vi "WPI_JoystickGetInfo.vi"(8 "error in (no error)":errorcluster, 11 "JoystickDevice":T1) -> (0 "error out":errorcluster, 2 "Joystick Info":T2)   [LabVIEW 2017]
doc: "Returns name, type, axis information, button and POV count for a joystick that you specify.\n\nThis software is licensed. Open the labview\\readme\\WPI Robotics Library Open Source License.txt file for more information."
uses:
  <vilib>/Rock Robotics/WPI/Joystick/WPI_Joystick Info.ctl
  <vilib>/Rock Robotics/WPI/Joystick/WPI_JoystickHID Types.ctl
  <vilib>/Rock Robotics/WPI/Joystick/WPI_JoystickXBox Types.ctl
  <vilib>/Rock Robotics/WPI/Joystick/WPI_JoystickAxis Types.ctl
  <vilib>/Rock Robotics/WPI/Joystick/WPI_JoystickDeviceEnum.ctl
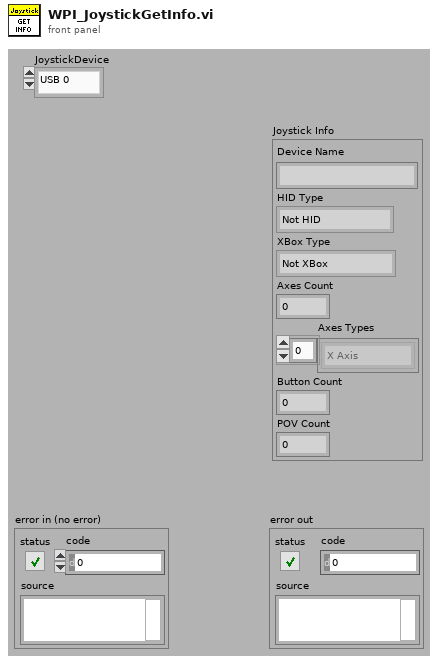
[diagram p1: front panel]
types:
  T1 = typedef "WPI_JoystickDeviceEnum.ctl" = enum16{"USB 0", "USB 1", "USB 2", "USB 3", "USB 4", "USB 5"}
  T2 = typedef "WPI_Joystick Info.ctl" = cluster{"Device Name":string, "HID Type":T3, "XBox Type":T4, "Axes Count":i32, "Axes Types":T5[], "Button Count":i32, "POV Count":i32}
  T3 = typedef "WPI_JoystickHID Types.ctl" = enum16{"Not HID", "HID Joystick", "HID Gamepad", "HID Driving Wheel", "HID Flightstick", "HID First Person"}
  T4 = typedef "WPI_JoystickXBox Types.ctl" = enum16{"Not XBox", "XBox Unknown", "XBox Gamepad", "XBox Wheel", "XBox Arcade Stick", "XBox Flight Stick", "XBox Dance Pad", "XBox Guitar", "XBox Drum Kit", "XBox Arcade Pad"}
  T5 = typedef "WPI_JoystickAxis Types.ctl" = enum16{"X Axis", "Y Axis", "Z Axis", "RxAxis", "RyAxis", "RzAxis", "Slider", "POV", "None", "L X Axis", "L Y Axis", "L Trigger", "R Trigger", "R X Axis", "R Y Axis"}
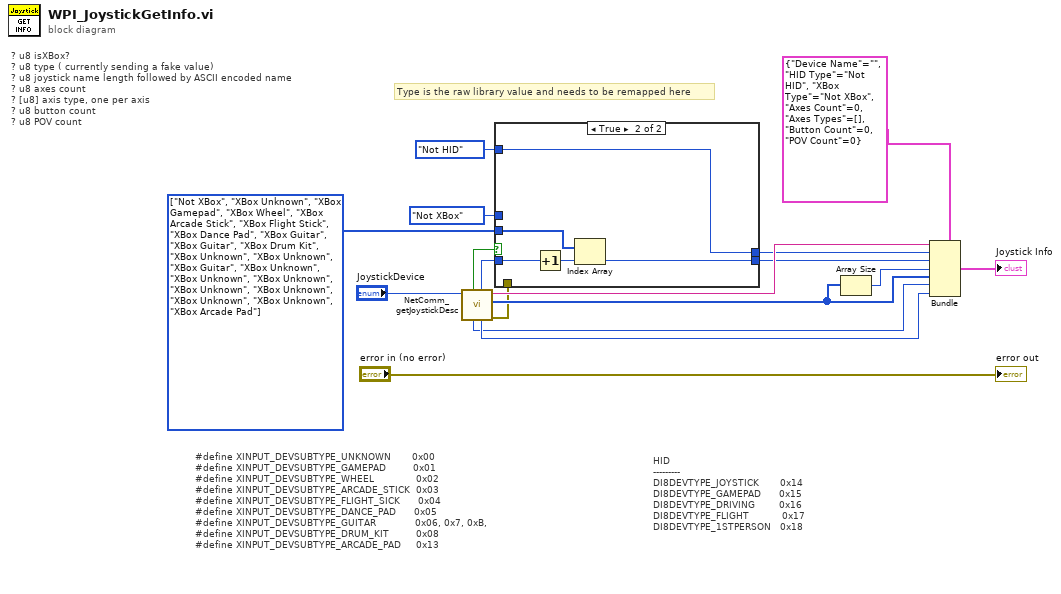
[diagram p0: block diagram]
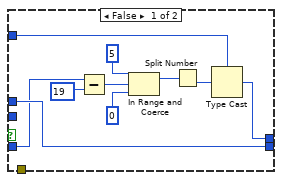
[diagram p2: hidden frame]
diagram:
  w2 = T4[] [enum."Not XBox", enum."XBox Unknown", enum."XBox Gamepad", enum."XBox Wheel", enum."XBox Arcade Stick", enum."XBox Flight Stick", enum."XBox Dance Pad", enum."XBox Guitar", enum."XBox Guitar", enum."XBox Drum Kit", enum."XBox Unknown", enum."XBox Unknown", enum."XBox Guitar", enum."XBox Unknown", enum."XBox Unknown", enum."XBox Unknown", enum."XBox Unknown", enum."XBox Unknown", enum."XBox Unknown", enum."XBox Unknown", enum."XBox Arcade Pad"] items=["Not XBox", "XBox Unknown", "XBox Gamepad", "XBox Wheel", "XBox Arcade Stick", "XBox Flight Stick", "XBox Dance Pad", "XBox Guitar", "XBox Drum Kit", "XBox Arcade Pad"]
  # "Type is the raw library value and needs to be remapped here"
  # "HID\n---------\nDI8DEVTYPE_JOYSTICK       0x14\nDI8DEVTYPE_GAMEPAD      0x15\nDI8DEVTYPE_DRIVING        0x16\nDI8DEVTYPE_FLIGHT           0x17\nDI8DEVTYPE_1STPERSON   0x18"
  # "#define XINPUT_DEVSUBTYPE_UNKNOWN       0x00\n#define XINPUT_DEVSUBTYPE_GAMEPAD         0x01\n#define XINPUT_DEVSUBTYPE_WHEEL              0x02\n#define XINPUT_DEVSUBTYPE_ARCADE_STICK  0x03\n#define XINPUT_DEVSUBTYPE_FLIGHT_SICK      0x04\n#define XINPUT_DEVSUBTYPE_DANCE_PAD      0x05\n#define XINPUT_DEVSUBTYPE_GUITAR             0x06, 0x7, 0xB, \n#define XINPUT_DEVSUBTYPE_DRUM_KIT         0x08\n#define XINPUT_DEVSUBTYPE_ARCADE_PAD     0x13"
  # "?\tu8 isXBox?\n?\tu8 type ( currently sending a fake value)\n?\tu8 joystick name length followed by ASCII encoded name\n?\tu8 axes count\n?\t[u8] axis type, one per axis\n?\tu8 button count\n?\tu8 POV count"
  n1 = call <vilib>:"NetComm_getJoystickDesc.vi"("Joystick Number"="JoystickDevice") -> ("error out"=w3:errorcluster, "Axis Types"=w9:u8[], "Name"=w15:string, "POV Count"=w13:u8, "Type"=w10:u8, "Button Count"=w12:u8, "Is XBox"=w11:bool)  [unwired: 4 in]
  n2 = case shown="True" w11 {
    tunnel: w10 -> [w24 w29]
    tunnel: [w25 w28] -> w7
    tunnel: [w26 w32] -> w6
    tunnel: WPI_JoystickXBox_Types."Not XBox" ("XBox Type") -> [w25 _]
    tunnel: WPI_JoystickHID_Types."Not HID" ("HID Type") -> [w27 w32]
    tunnel: w3 -> [_ _]
    tunnel: w2 -> [_ w30]
    frame False {
      n3 = Subtract(x=w24, y=19) -> (x-y=w22:i32)
      n4 = In Range and Coerce(upper limit=5, x=w22, lower limit=0) -> (coerced(x)=w19:i32)  [unwired: 1 out]
      n5 = Split Number(x=w19) -> (lo(x)=w18:u16)  [unwired: 1 out]
      n6 = Type Cast(type=w27, x=w18) -> (*(type *) &x=w26:T3)
    }
    frame True {
      n7 = Increment(x=w29) -> (x+1=w31:u8)
      n8 = Index Array(array=w30, index=w31) -> (element=w28:T4)
    }
  }
  n9 = Array Size(array=w9) -> (size(s)=w8:i32)
  n10 = Bundle(cluster=T2 {"Device Name"="", "HID Type"=enum."Not HID", "XBox Type"=enum."Not XBox", "Axes Count"=0, "Axes Types"=[], "Button Count"=0, "POV Count"=0} ("Joystick Info"), "Device Name"=w15, "HID Type"=w6, "XBox Type"=w7, "Axes Count"=w8, "Axes Types"=w9, "Button Count"=w12, "POV Count"=w13) -> (→"Joystick Info":T2)
  "error out" <- "error in (no error)"
